vi "comms_Serial_Open.vi"(6 "Send Init Comm?":bool, 8 "error in (no error)":errorcluster, 9 "Serial Settings in":T1, 11 "VISA Refnum in":refnum<visa-resource-name>) -> (0 "error out":errorcluster, 2 "Data Out":string, 3 "VISA Refnum out":refnum<visa-resource-name>)   [LabVIEW 2018]
uses:
  <vilib>/Instr/_visa.llb/VISA Configure Serial Port (Instr).vi
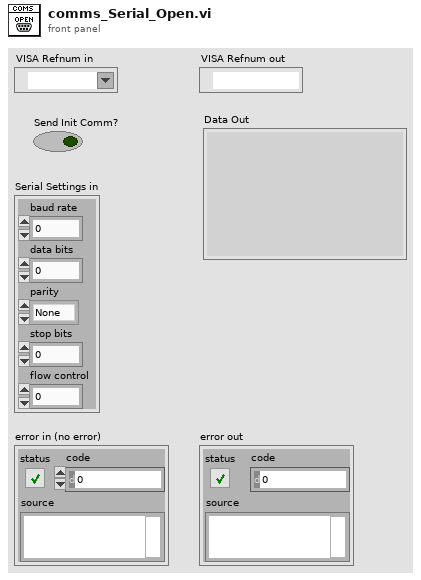
[diagram p1: front panel]
types:
  T1 = cluster{"baud rate":u32, "data bits":u16, "parity":enum16{"None", "Odd", "Even", "Mark", "Space"}, "stop bits":u16, "flow control":u16}
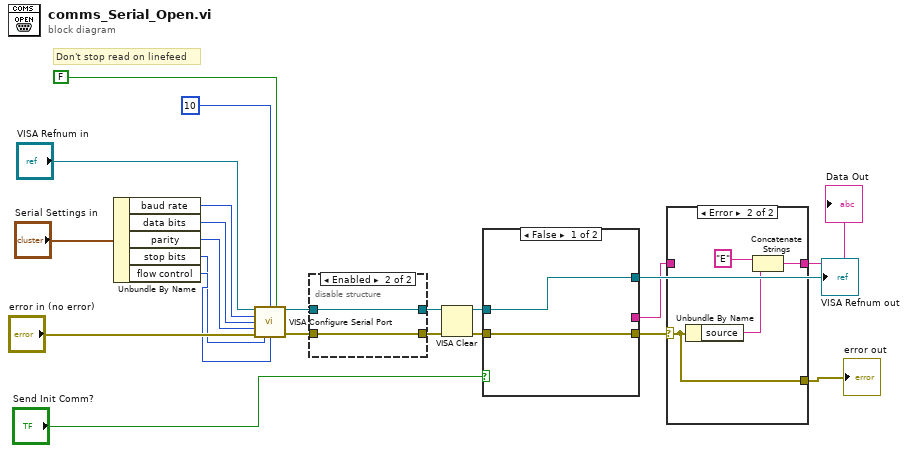
[diagram p0: block diagram]
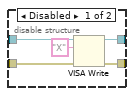
[diagram p2: hidden frame]
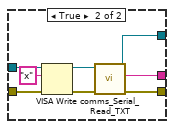
[diagram p3: hidden frame]
diagram:
  # "Don't stop read on linefeed"
  n1 = Unbundle By Name("Serial Settings in") -> ("baud rate"=w17:u32, "data bits"=w16:u16, "parity"=w15:enum16{"None", "Odd", "Even", "Mark", "Space"}, "stop bits"=w14:u16, "flow control"=w20:u16)
  n2 = call-poly "VISA Configure Serial Port"("VISA resource name"="VISA Refnum in", "termination char\n(0xA = '\\n' = LF)"=u8 10 ("Termination Character"), "Enable Termination\nChar (T)"=FALSE ("End Read on Termination Character?"), "baud rate (9600)"=w17, "data bits (8)"=w16, "parity (0:none)"=w15, "error in (no error)"="error in (no error)", "stop bits (10: 1 bit)"=w14, "flow control (0:none)"=w20) -> ("VISA resource name out"=w7:refnum<visa-resource-name>, "error out"=w6:errorcluster)  [unwired: 1 in, 4 out]
  n3 = disable-structure shown="Enabled" {
    disable-tunnel: w7 -> [w27 w29]
    disable-tunnel: w6 -> [w26 w28]
    disable-tunnel: [w24 w28] -> w5
    disable-tunnel: [w23 w29] -> w4
    frame Disabled {
      n4 = VISA Write(VISA resource name=w27, write buffer="X", error in (no error)=w26) -> (VISA resource name out=w23:refnum<visa-resource-name>, error out=w24:errorcluster)  [unwired: 1 out]
    }
    frame Enabled {
    }
  }
  n5 = VISA Clear(VISA resource name=w4, error in (no error)=w5) -> (VISA resource name out=w2:refnum<visa-resource-name>, error out=w3:errorcluster)
  n6 = case shown="False" "Send Init Comm?" {
    tunnel: [w31 w39] -> w12
    tunnel: [w30 w38] -> w11
    tunnel: [_ w37] -> w9
    tunnel: w3 -> [w30 w36]
    tunnel: w2 -> [w31 w34]
    frame False {
    }
    frame True {
      n7 = VISA Write(VISA resource name=w34, write buffer="x", error in (no error)=w36) -> (VISA resource name out=w33:refnum<visa-resource-name>, error out=w35:errorcluster)  [unwired: 1 out]
      n8 = call "comms_Serial_Read_TXT.vi"("error in"=w35, "VISA resource in"=w33) -> ("error out"=w38:errorcluster, "Data Out"=w37:string, "VISA resource Out"=w39:refnum<visa-resource-name>)  [unwired: 6 in, 1 out]
    }
  }
  "VISA Refnum out" <- w12
  n9 = case shown="Error" w11 {
    selector: w11 -> [w41 w45]
    tunnel: [w41 w45] -> w10
    tunnel: w9 -> [w40 _]
    tunnel: [w40 w44] -> w8
    frame No Error {
    }
    frame Error {
      n10 = Unbundle By Name(w45) -> ("source"=w43:string)
      n11 = Concatenate Strings("E", w43) -> (w44:string)
    }
  }
  "error out" <- w10
  "Data Out" <- w8
